vi "SetWindowPos.vi"(6 "Flags":T1, 7 "hWndInsertAfterALT\n(HWND_TOP)":T2(ring), 8 "error in (no error)":errorcluster, 9 "Metrics (0,0,0,0)":cluster{"X":i32, "Y":i32, "cx":i32, "cy":i32}, 10 "hWndInsertAfter\n(NULL - use ALT)":T3, 11 "hWnd (NULL)":T3) -> (0 "error out":errorcluster, 3 "dup hWnd":T3)   [LabVIEW 2011]
doc: "SetWindowPos\nThe SetWindowPos function changes the size, position, and Z order of a child, pop-up, or top-level window. Child, pop-up, and top-level windows are ordered according to their appearance on the screen. The topmost window receives the highest rank and is the first window in the Z order. \n\nBOOL SetWindowPos(\n HWND hWnd, // handle to window\n HWND hWndInsertAfter, // placement-order handle\n int X, // horizontal position\n int Y, // vertical position\n int cx, // width\n int cy, // height\n UINT uFlags // window-positioning options\n);\nParameters\nhWnd \n[in] Handle to the window. \nhWndInsertAfter \n[in] Handle to the window to precede the positioned window in the Z order. This parameter must be a window handle or one of the following values. Value Meaning \nHWND_BOTTOM Places the window at the bottom of the Z order. If the hWnd parameter identifies a topmost window, the window loses its topmost status and is placed at the bottom of all other windows. \nHWND_NOTOPMOST Places the window above all non-topmost windows (that is, behind all topmost windows). This flag has no effect if the window is already a non-topmost window. \nHWND_TOP Places the window at the top of the Z order. \nHWND_TOPMOST Places the window above all non-topmost windows. The window maintains its topmost position even when it is deactivated. \n\n\nFor more information about how this parameter is used, see the following Remarks section. \n\nX \n[in] Specifies the new position of the left side of the window, in client coordinates. \nY \n[in] Specifies the new position of the top of the window, in client coordinates. \ncx \n[in] Specifies the new width of the window, in pixels. \ncy \n[in] Specifies the new height of the window, in pixels. \nuFlags \n[in] Specifies the window sizing and positioning flags. This parameter can be a combination of the following values. Value Meaning \nSWP_ASYNCWINDOWPOS If the calling thread and the thread that owns the window are attached to different input queues, the system posts the request to the thread that owns the window. This prevents the calling thread from blocking its execution while other threads process the request. \nSWP_DEFERERASE Prevents generation of the WM_SYNCPAINT message. \nSWP_DRAWFRAME Draws a frame (defined in the window's class description) around the window. \nSWP_FRAMECHANGED Applies new frame styles set using the SetWindowLong function. \nSends a WM_NCCALCSIZE message to the window, even if the window's size is not being changed. If this flag is not specified, WM_NCCALCSIZE is sent only when the window's size is being changed.\n \nSWP_HIDEWINDOW Hides the window. \nSWP_NOACTIVATE Does not activate the window. If this flag is not set, the window is activated and moved to the top of either the topmost or non-topmost group (depending on the setting of the hWndInsertAfter parameter). \nSWP_NOCOPYBITS Discards the entire contents of the client area. If this flag is not specified, the valid contents of the client area are saved and copied back into the client area after the window is sized or repositioned. \nSWP_NOMOVE Retains the current position (ignores the X and Y parameters). \nSWP_NOOWNERZORDER Does not change the owner window's position in the Z order. \nSWP_NOREDRAW Does not redraw changes. If this flag is set, no repainting of any kind occurs. This applies to the client area, the nonclient area (including the title bar and scroll bars), and any part of the parent window uncovered as a result of the window being moved. When this flag is set, the application must explicitly invalidate or redraw any parts of the window and parent window that need redrawing. \nSWP_NOREPOSITION Same as the SWP_NOOWNERZORDER flag. \nSWP_NOSENDCHANGING Prevents the window from receiving the WM_WINDOWPOSCHANGING message. \nSWP_NOSIZE Retains the current size (ignores the cx and cy parameters). \nSWP_NOZORDER Retains the current Z order (ignores the hWndInsertAfter parameter). \nSWP_SHOWWINDOW Displays the window. \n\n\nReturn Values\nIf the function succeeds, the return value is nonzero.\n\nIf the function fails, the return value is zero. To get extended error information, call GetLastError. \n\nRemarks\nIf the SWP_SHOWWINDOW or SWP_HIDEWINDOW flag is set, the window cannot be moved or sized. \n\nIf you have changed certain window data using SetWindowLong, you must call SetWindowPos to have the changes take effect. Use the following combination for uFlags: SWP_NOMOVE | SWP_NOSIZE | SWP_NOZORDER | SWP_FRAMECHANGED. \n\nA window can be made a topmost window either by setting the hWndInsertAfter parameter to HWND_TOPMOST and ensuring that the SWP_NOZORDER flag is not set, or by setting a window's position in the Z order so that it is above any existing topmost windows. When a non-topmost window is made topmost, its owned windows are also made topmost. Its owners, however, are not changed. \n\nIf neither the SWP_NOACTIVATE nor SWP_NOZORDER flag is specified (that is, when the application requests that a window be simultaneously activated and its position in the Z order changed), the value specified in hWndInsertAfter is used only in the following circumstances: \n\nNeither the HWND_TOPMOST nor HWND_NOTOPMOST flag is specified in hWndInsertAfter. \nThe window identified by hWnd is not the active window. \nAn application cannot activate an inactive window without also bringing it to the top of the Z order. Applications can change an activated window's position in the Z order without restrictions, or it can activate a window and then move it to the top of the topmost or non-topmost windows. \n\nIf a topmost window is repositioned to the bottom (HWND_BOTTOM) of the Z order or after any non-topmost window, it is no longer topmost. When a topmost window is made non-topmost, its owners and its owned windows are also made non-topmost windows. \n\nA non-topmost window can own a topmost window, but the reverse cannot occur. Any window (for example, a dialog box) owned by a topmost window is itself made a topmost window, to ensure that all owned windows stay above their owner. \n\nIf an application is not in the foreground, and should be in the foreground, it must call the SetForegroundWindow function."
uses:
  hWnd.ctl
  user32.dll
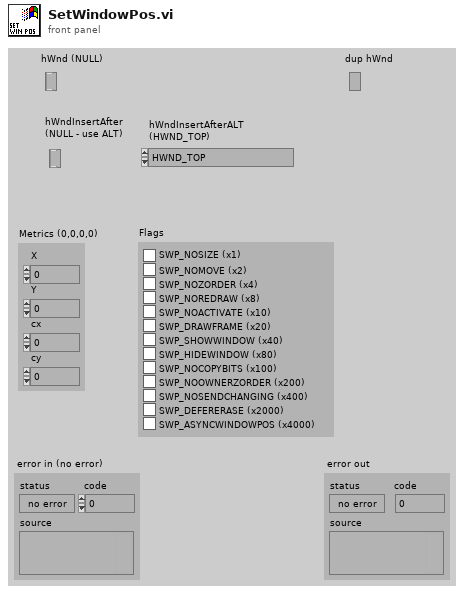
[diagram p1: front panel]
types:
  T1 = cluster{"SWP_NOSIZE (x1)":bool, "SWP_NOMOVE (x2)":bool, "SWP_NOZORDER (x4)":bool, "SWP_NOREDRAW (x8)":bool, "SWP_NOACTIVATE (x10)":bool, "SWP_DRAWFRAME (x20)":bool, "SWP_SHOWWINDOW (x40)":bool, "SWP_HIDEWINDOW (x80)":bool, "SWP_NOCOPYBITS (x100)":bool, "SWP_NOOWNERZORDER (x200)":bool, "SWP_NOSENDCHANGING (x400)":bool, "SWP_DEFERERASE (x2000)":bool, "SWP_ASYNCWINDOWPOS (x4000)":bool}
  T2 = enum16{"HWND_TOP", "HWND_BOTTOM", "HWND_TOPMOST", "HWND_NOTOPMOST"}
  T3 = typedef "hWnd.ctl" = refnum<k1>
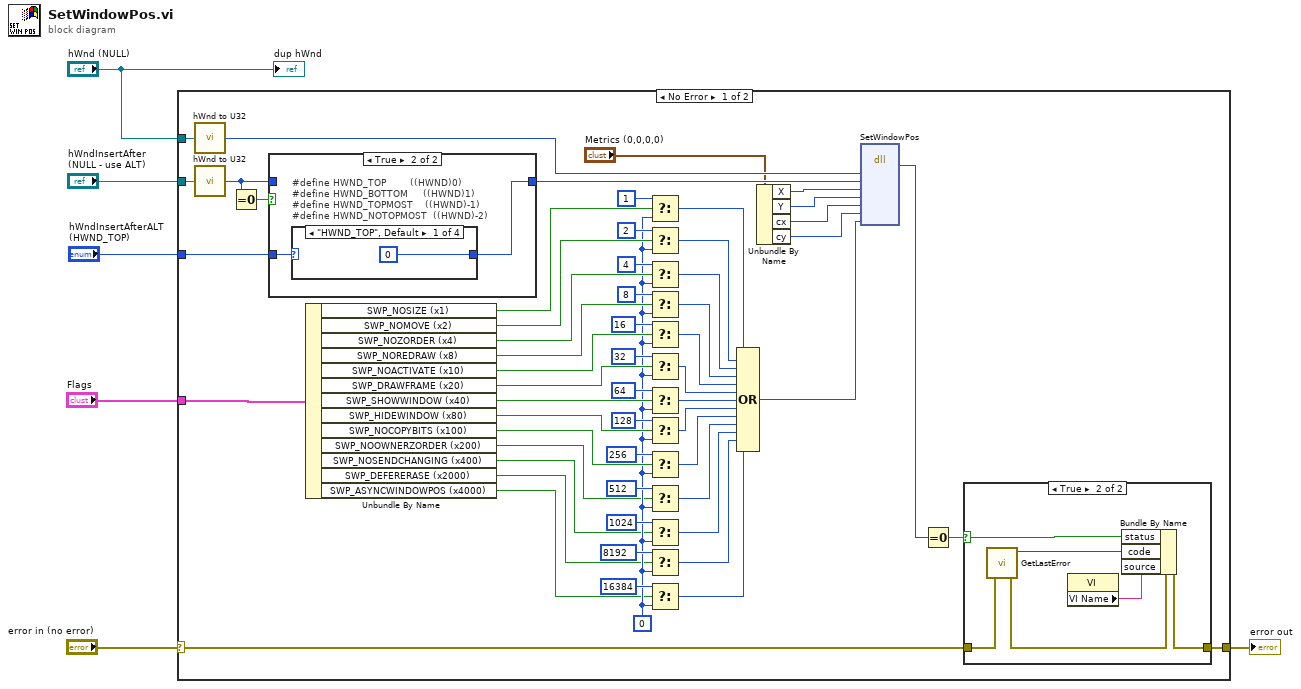
[diagram p0: block diagram]
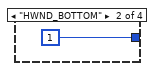
[diagram p4: hidden frame]
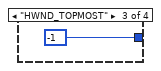
[diagram p5: hidden frame]
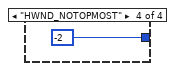
[diagram p6: hidden frame]
diagram:
  n1 = case shown="No Error" "error in (no error)" {
    selector: "error in (no error)" -> [w7 w79]
    tunnel: [w9 w79] -> w5
    tunnel: "hWnd (NULL)" -> [w63 _]
    tunnel: "hWndInsertAfter\n(NULL - use ALT)" -> [w61 _]
    tunnel: "hWndInsertAfterALT\n(HWND_TOP)" -> [w57 _]
    tunnel: "Flags" -> [w37 _]
    frame No Error {
      w23 = u32 0 ("left")
      n2 = call "hWnd to U32.vi"("hWnd"=w63) -> ("hWnd"=w62:u32)  [unwired: 4 out]
      n3 = call "hWnd to U32.vi"("hWnd"=w61) -> ("hWnd"=w59:u32)  [unwired: 4 out]
      n4 = Equal To 0?(x=w59) -> (x = 0?=w60:bool)
      n5 = case shown="True" w60 {
        tunnel: w59 -> [w72 _]
        tunnel: [w72 w73] -> w58
        tunnel: w57 -> [_ w74]
        frame False {
        }
        frame True {
          n6 = case "#define HWND_TOP        ((HWND)0)\n#define HWND_BOTTOM     ((HWND)1)\n#define HWND_TOPMOST    ((HWND)-1)\n#define HWND_NOTOPMOST  ((HWND)-2)" shown="\"HWND_TOP\", Default" w74 {
            tunnel: [u32 0 u32 1 -1 -2] -> w73
            frame "HWND_TOP", Default {
            }
            frame "HWND_BOTTOM" {
            }
            frame "HWND_TOPMOST" {
            }
            frame "HWND_NOTOPMOST" {
            }
          }
        }
      }
      n7 = Unbundle By Name(w37) -> ("SWP_NOSIZE (x1)"=w36:bool, "SWP_NOMOVE (x2)"=w35:bool, "SWP_NOZORDER (x4)"=w34:bool, "SWP_NOREDRAW (x8)"=w33:bool, "SWP_NOACTIVATE (x10)"=w32:bool, "SWP_DRAWFRAME (x20)"=w31:bool, "SWP_SHOWWINDOW (x40)"=w30:bool, "SWP_HIDEWINDOW (x80)"=w29:bool, "SWP_NOCOPYBITS (x100)"=w28:bool, "SWP_NOOWNERZORDER (x200)"=w18:bool, "SWP_NOSENDCHANGING (x400)"=w17:bool, "SWP_DEFERERASE (x2000)"=w16:bool, "SWP_ASYNCWINDOWPOS (x4000)"=w15:bool)
      n8 = Select(t=u32 1 ("left"), s=w36, f=w23) -> (s? t:f=w55:u32)
      n9 = Select(t=u32 2 ("left"), s=w35, f=w23) -> (s? t:f=w53:u32)
      n10 = Select(t=u32 4 ("left"), s=w34, f=w23) -> (s? t:f=w51:u32)
      n11 = Select(t=u32 8 ("left"), s=w33, f=w23) -> (s? t:f=w49:u32)
      n12 = Select(t=u32 16 ("left"), s=w32, f=w23) -> (s? t:f=w43:u32)
      n13 = Select(t=u32 32 ("left"), s=w31, f=w23) -> (s? t:f=w42:u32)
      n14 = Select(t=u32 64 ("left"), s=w30, f=w23) -> (s? t:f=w41:u32)
      n15 = Select(t=u32 128 ("left"), s=w29, f=w23) -> (s? t:f=w40:u32)
      n16 = Select(t=u32 256 ("left"), s=w28, f=w23) -> (s? t:f=w39:u32)
      n17 = Select(t=u32 512 ("left"), s=w18, f=w23) -> (s? t:f=w22:u32)
      n18 = Select(t=u32 1024 ("left"), s=w17, f=w23) -> (s? t:f=w21:u32)
      n19 = Select(t=u32 8192 ("left"), s=w16, f=w23) -> (s? t:f=w20:u32)
      n20 = Select(t=u32 16384 ("left"), s=w15, f=w23) -> (s? t:f=w19:u32)
      n21 = Compound Arithmetic op=OR(w55, w53, w51, w49, w43, w42, w41, w40, w39, w22, w21, w20, w19) -> (w38:u32)
      n22 = Unbundle By Name("Metrics (0,0,0,0)") -> ("X"=w13:i32, "Y"=w12:i32, "cx"=w11:i32, "cy"=w10:i32)
      n23 = dll-call lib="user32.dll" fn="SetWindowPos"("hWnd"=w62, "hWndInsertAfter"=w58, "X"=w13, "Y"=w12, "cx"=w11, "cy"=w10, "fuFlags"=w38) -> ("error"=w64:i32)  [unwired: 10 in, 2 out]
      n24 = Equal To 0?(x=w64) -> (x = 0?=w8:bool)
      n25 = case shown="True" w8 {
        selector: w8 -> [_ w66]
        tunnel: w7 -> [w65 w70]
        tunnel: [w65 w71] -> w9
        frame False {
        }
        frame True {
          n26 = call "GetLastError.vi"("error in (no error)"=w70) -> ("error out"=w69:errorcluster, "CODE"=w68:i32)  [unwired: 5 out]
          n27 = property class="VI"() -> ("VI Name"=w67:string)  [unwired: 2 in, 2 out]
          n28 = Bundle By Name(cluster=w69, "status"=w66, "code"=w68, "source"=w67) -> (w71:errorcluster)
        }
      }
    }
    frame Error {
    }
  }
  "error out" <- w5
  "dup hWnd" <- "hWnd (NULL)"
